vi "gyro_binary_dataset_to_scaled_xyz.vi"(0 "binarySet":u8[](array[numeric])) -> (2 "x axis value":dbl, 3 "y axis value":dbl, 4 "z axis value":dbl)   [LabVIEW 2017]
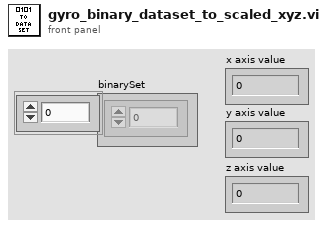
[diagram p1: front panel]
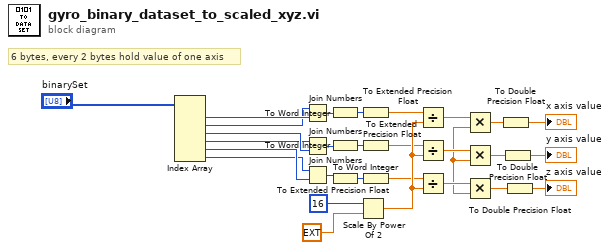
[diagram p0: block diagram]
diagram:
  # "6 bytes, every 2 bytes hold value of one axis"
  n1 = Index Array(array="binarySet") -> (element #1=w29:u8, element #2=w28:u8, element #3=w27:u8, element #4=w26:u8, element #5=w25:u8, element #6=w24:u8)  [unwired: 6 in]
  n2 = Join Numbers(hi=w28, lo=w29) -> ((hi.lo)=w23:u16)
  n3 = Join Numbers(hi=w26, lo=w27) -> ((hi.lo)=w22:u16)
  n4 = Join Numbers(hi=w24, lo=w25) -> ((hi.lo)=w21:u16)
  n5 = To Word Integer(number=w23) -> (16bit integer=w9:i16)
  n6 = To Word Integer(number=w22) -> (16bit integer=w10:i16)
  n7 = To Word Integer(number=w21) -> (16bit integer=w12:i16)
  n8 = Scale By Power Of 2(n=i16 16, x=ext 1.0) -> (x*2^n=w15:ext)
  n9 = To Extended Precision Float(1:w9) -> (0:w8:ext)
  n10 = To Extended Precision Float(1:w10) -> (0:w11:ext)
  n11 = To Extended Precision Float(1:w12) -> (0:w13:ext)
  n12 = Divide(x=w8, y=w15) -> (x/y=w18:ext)
  n13 = Divide(x=w11, y=w15) -> (x/y=w17:ext)
  n14 = Divide(x=w13, y=w15) -> (x/y=w16:ext)
  n15 = Multiply(x=w17) -> (y=w14:ext, x*y=w5:ext)
  n16 = Multiply(x=w18, y=w14) -> (x*y=w4:ext)
  n17 = Multiply(x=w16, y=w14) -> (x*y=w6:ext)
  n18 = To Double Precision Float(number=w4) -> (double precision float=→"x axis value":dbl)
  n19 = To Double Precision Float(number=w5) -> (double precision float=→"y axis value":dbl)
  n20 = To Double Precision Float(number=w6) -> (double precision float=→"z axis value":dbl)
